vi "Clear No Tag Error.vi"(8 "error in (no error)":errorcluster) -> (0 "error out":errorcluster)   [LabVIEW 2014, in "Scan Engine editor node.lvclass"]
uses:
  Scan Engine editor node.lvclass
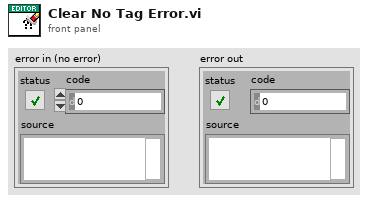
[diagram p1: front panel]
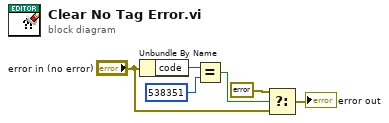
[diagram p0: block diagram]
diagram:
  n1 = Unbundle By Name("error in (no error)") -> ("code"=w4:i32)
  n2 = Equal?(x=w4, y=538351 ("code")) -> (x = y?=w5:bool)
  n3 = Select(t=errorcluster {"status"=FALSE, "code"=0, "source"=""} ("f"), s=w5, f="error in (no error)") -> (s? t:f=→"error out":errorcluster)
